vi "UpdateImageDisplayGraph.vi"(10 "ImageInfo":T1, 11 "IntensityGraph in":refnum<vi>) -> ()   [LabVIEW 2017]
uses:
  Types/ImageInfo.ctl
  <vilib>/express/express arith-compare/Formula/XNode/ExpressFormulaBlockNode.xnode
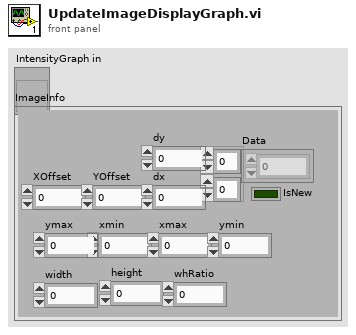
[diagram p1: front panel]
types:
  T1 = typedef "ImageInfo.ctl" = cluster{"IsNew":bool, "Data":dbl[][], "XOffset":dbl, "YOffset":dbl, "dy":dbl, "dx":dbl, "xmin":dbl, "xmax":dbl, "ymin":dbl, "ymax":dbl, "width":dbl, "height":dbl, "whRatio":dbl}
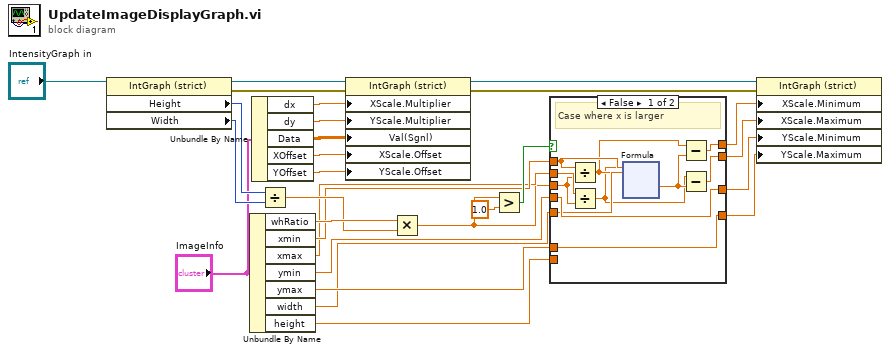
[diagram p0: block diagram]
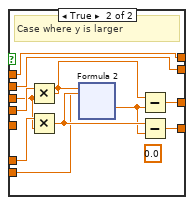
[diagram p2: hidden frame]
diagram:
  n1 = property class="IntGraph (strict)"(reference="IntensityGraph in") -> (reference out=w4:refnum<vi>, error out=w5:errorcluster, "Height"=w27:u32, "Width"=w26:u32)  [unwired: 1 in]
  n2 = Unbundle By Name("ImageInfo") -> ("whRatio"=w13:dbl, "xmin"=w11:dbl, "xmax"=w10:dbl, "ymin"=w9:dbl, "ymax"=w8:dbl, "width"=w1:dbl, "height"=w6:dbl)
  n3 = Unbundle By Name("ImageInfo") -> ("dx"=w21:dbl, "dy"=w20:dbl, "Data"=w19:dbl[][], "XOffset"=w3:dbl, "YOffset"=w2:dbl)
  n4 = Divide(x=w27, y=w26) -> (x/y=w12:dbl)
  n5 = property class="IntGraph (strict)"(reference=w4, error in=w5, "XScale.Multiplier"=w21, "YScale.Multiplier"=w20, "Val(Sgnl)"=w19, "XScale.Offset"=w3, "YScale.Offset"=w2) -> (reference out=w23:refnum<vi>, error out=w22:errorcluster)
  n6 = Multiply(x=w13, y=w12) -> (x*y=w7:dbl)
  n7 = Greater?(x=w7, y=1.0) -> (0:w24:bool)
  n8 = case shown="False" w24 {
    tunnel: [w35 w61] -> w18
    tunnel: [w37 w55] -> w16
    tunnel: [w34 w60] -> w17
    tunnel: [w36 w56] -> w15
    tunnel: w11 -> [w32 w61]
    tunnel: w10 -> [w39 w60]
    tunnel: w9 -> [w37 w64]
    tunnel: w8 -> [w36 w63]
    tunnel: w7 -> [w38 w62]
    tunnel: w6 -> [_ w57]
    tunnel: w1 -> [w33 _]
    frame False {
      # "Case where x is larger"
      n9 = Divide(x=w32, y=w38) -> (x/y=w30:dbl)
      n10 = Divide(x=w39, y=w38) -> (x/y=w29:dbl)
      n11 = xnode "Formula"("min"=w32, "l"=w33, "minR"=w30, "maxR"=w29) -> ("Result"=w31:dbl)  [unwired: 1 in, 1 out]
      n12 = Subtract(x=w30, y=w31) -> (x-y=w35:dbl)
      n13 = Subtract(x=w29, y=w31) -> (x-y=w34:dbl)
    }
    frame True {
      (unwired) 0.0 ("Y Scale.Offset and Multiplier:Offset")
      # "Case where y is larger"
      n14 = Multiply(x=w64, y=w62) -> (x*y=w59:dbl)
      n15 = Multiply(x=w63, y=w62) -> (x*y=w58:dbl)
      n16 = xnode "Formula 2"("min"=w59, "max"=w58, "l"=w57) -> ("Result"=w54:dbl)  [unwired: 1 in, 1 out]
      n17 = Subtract(x=w59, y=w54) -> (x-y=w55:dbl)
      n18 = Subtract(x=w58, y=w54) -> (x-y=w56:dbl)
    }
  }
  n19 = property class="IntGraph (strict)"(reference=w23, error in=w22, "XScale.Minimum"=w18, "XScale.Maximum"=w17, "YScale.Minimum"=w16, "YScale.Maximum"=w15) -> ()  [unwired: 2 out]
